vi "Memory.Pointer.Write.Safe.0D.I8.vi"(8 "error in (no error)":errorcluster, 10 "value":i8, 11 "pointer in":refnum<class "Memory.Pointer.lvclass">) -> (0 "error out":errorcluster, 2 "value":i8, 3 "pointer out":refnum<class "Memory.Pointer.lvclass">)   [LabVIEW 2016, in "Memory Manager.lvlib" / "Memory.Pointer.lvclass"]
doc: "Writes <b>count</b> elements from the provided <b>buffer</b> to the address specified by <b>pointer</b>.\n\n<b>Note:</b> This VI is <b>safe</b>.\n\nSafe means that this function evaluates the size parameter of <b>pointer</b> to ensure that is inbounds of allocated memory before peforming a memory read/write. Reading/writing more data to a pointer than it has allocated can corrupt or crash LabVIEW."
uses:
  Memory.Pointer.lvclass
  Memory.Pointer.lvclass/Memory.Pointer.ctl
  Accessors/Get Address.vi
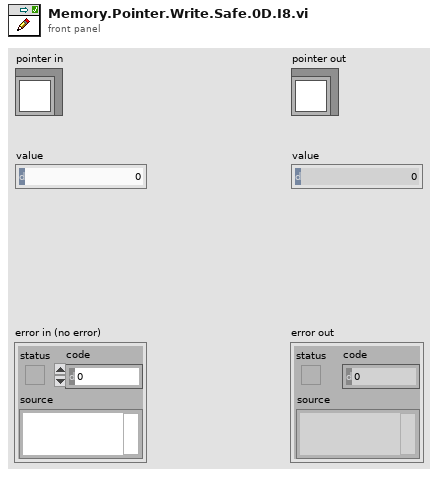
[diagram p1: front panel]
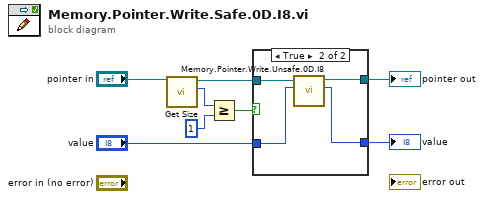
[diagram p0: block diagram]
diagram:
  n1 = call "Get Size.vi"("Pointer in"="pointer in") -> ("size"=w7:u64, "Pointer out"=w4:refnum<class "Memory.Pointer.lvclass">)  [unwired: 8 in, 1 out]
  n2 = Greater Or Equal?(x=w7, y=u64 1) -> (x >= y?=w5:bool)
  n3 = case shown="True" w5 {
    tunnel: w4 -> [w10 w14]
    tunnel: [w10 w13] -> w3
    tunnel: [w9 w12] -> w2
    tunnel: "value" -> [w9 w11]
    frame False {
    }
    frame True {
      n4 = call "Memory.Pointer.Write.Unsafe.0D.I8.vi"("value"=w11, "pointer in"=w14) -> ("value"=w12:i8, "pointer out"=w13:refnum<class "Memory.Pointer.lvclass">)  [unwired: 7 in, 1 out]
    }
  }
  "pointer out" <- w3
  "value" <- w2
